vi "FreeTracker.vi"(0 "trackerInstance":u64) -> ()   [LabVIEW 2011]
uses:
  cudatrack-debug.dll
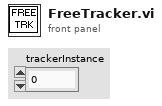
[diagram p1: front panel]
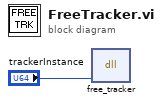
[diagram p0: block diagram]
diagram:
  n1 = dll-call lib="D:/jcnossen1/cudaqi-tracker/cudatrack/cudatrack-debug.dll" fn="free_tracker"("trackerInstance"="trackerInstance") -> ()  [unwired: 5 in, 2 out]
